vi "Main - Stock Ticker.vi"() -> ()   [LabVIEW 2011]
doc: "Main VI for a stock ticker application.\n\nInstructions:\n1) Select the data source.\n2) Enter the stock's symbol. Note that, for every letter typed, an HTTP query is sent (this is a trade-off between expecting the user to know the quotes and using a local list of quotes).\n3) Press the add button to add the ticker to the stock table.\n4) Press the delete button to delete the ticker the stock table.\n5) The delay between quote refresh is adjustable.\n6) The stop button will stop the application."
panel:
  in  "Delete":bool
  out "Stock Table":string[][](table)
  in  "Source":enum16{"Google", "Yahoo"}(ring)
  out "Consumer":bool
  out "Producer":bool
  out "Timer":bool
  out "Updating":bool
  in  "Refresh":i32=5 caption="Refresh rate [s]" min=0
  in  "Stop":bool
  in  "Add":bool
  in  "Stock Data":T1
  out "error out":errorcluster
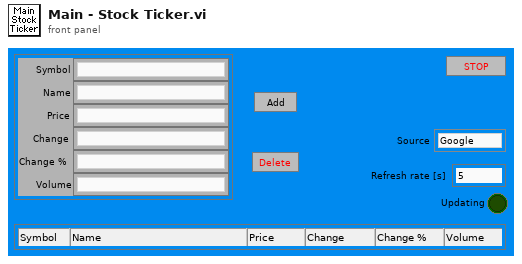
[diagram p1: front panel]
types:
  T1 = cluster{"Symbol":string, "Name":string, "Price":string, "Change":string, "Change %":string, "Volume":string}
  T2 = typedef "Queue RefNum" = refnum<k1>
  T3 = enum16{"Symbol", "Name", "Price", "Change", "Change %", "Volume"}
  T4 = typedef "Stock Data Control.ctl" = cluster{"Symbol":string, "Name":string, "Price":string, "Change":string, "Change %":string, "Volume":string}
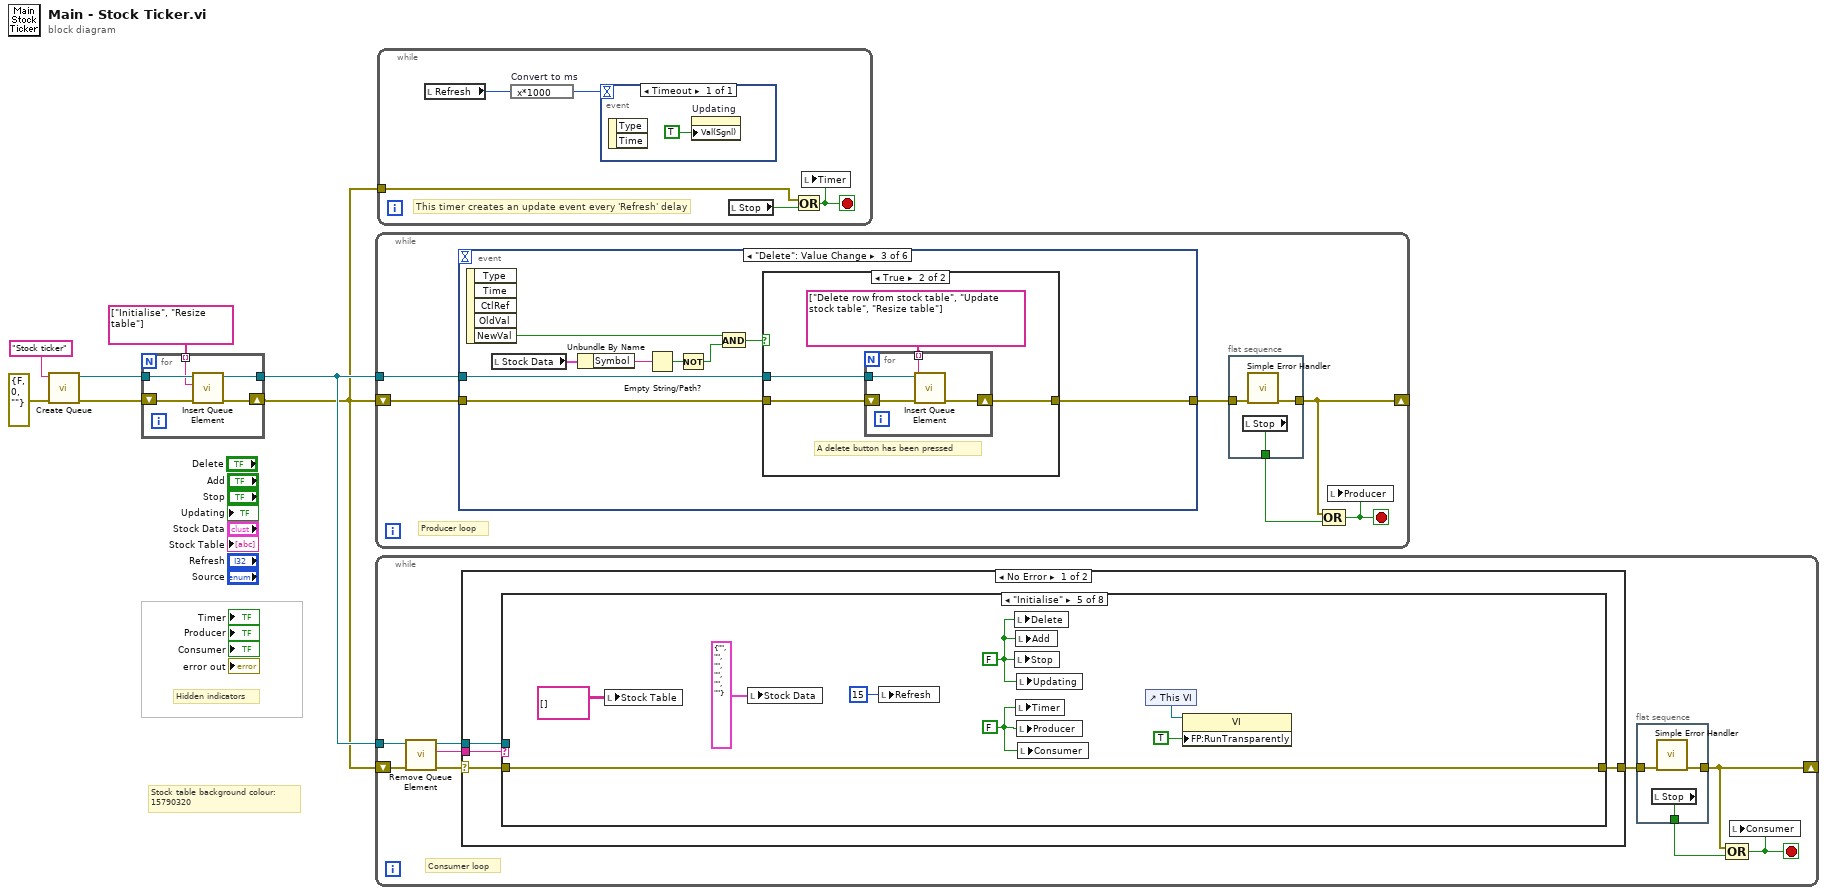
[diagram p0: block diagram]
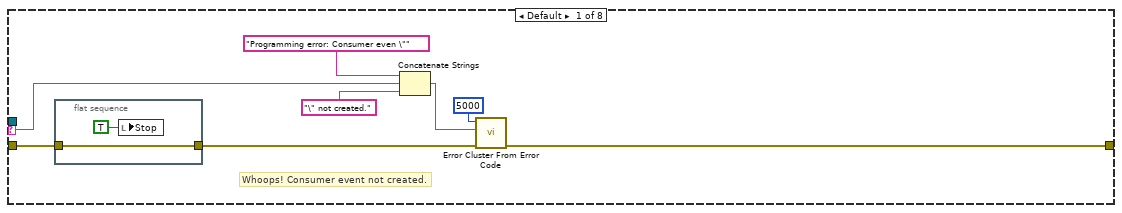
[diagram p2: hidden frame]
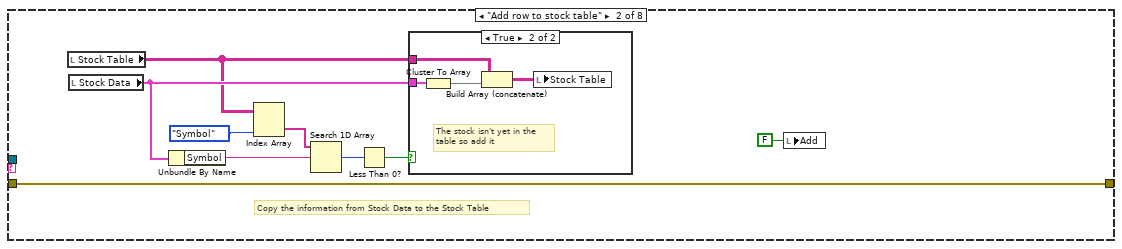
[diagram p3: hidden frame]
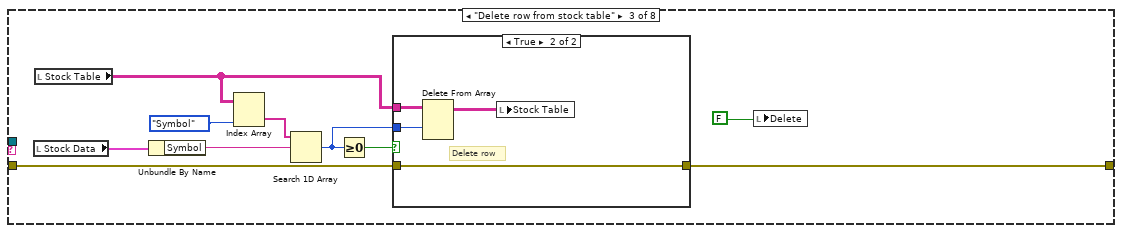
[diagram p5: hidden frame]
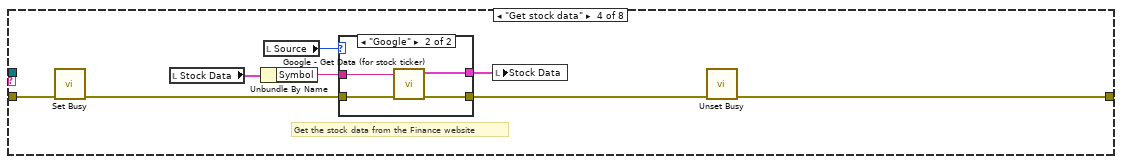
[diagram p7: hidden frame]
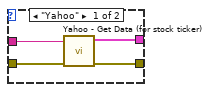
[diagram p8: hidden frame]
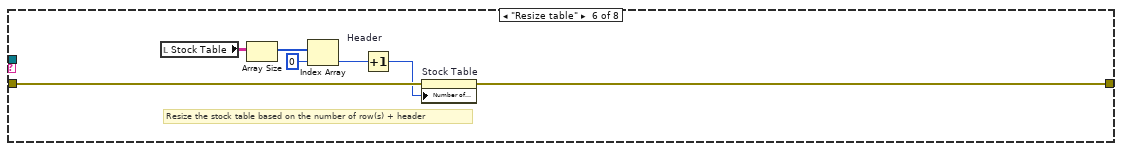
[diagram p9: hidden frame]
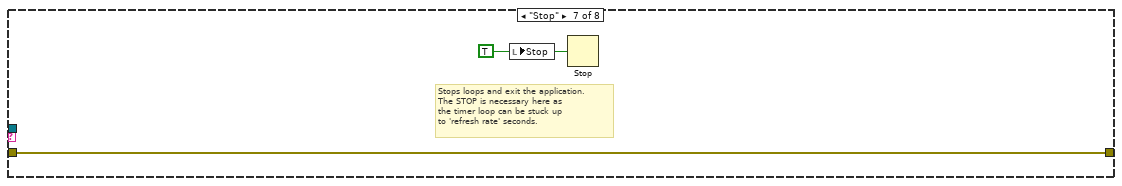
[diagram p10: hidden frame]
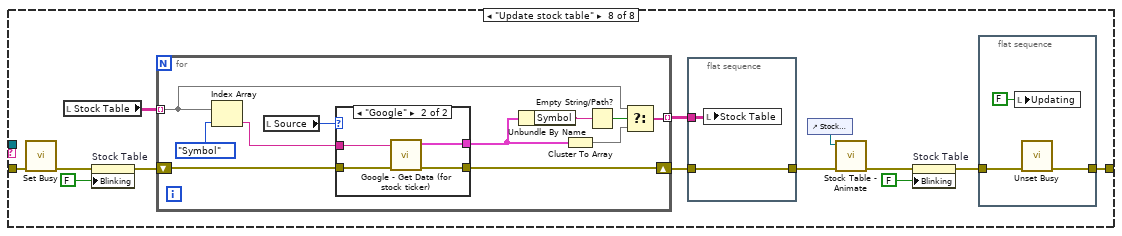
[diagram p11: hidden frame]
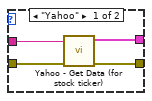
[diagram p12: hidden frame]
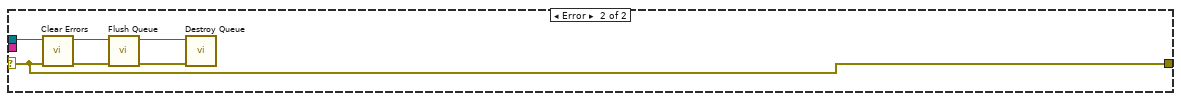
[diagram p13: hidden frame]
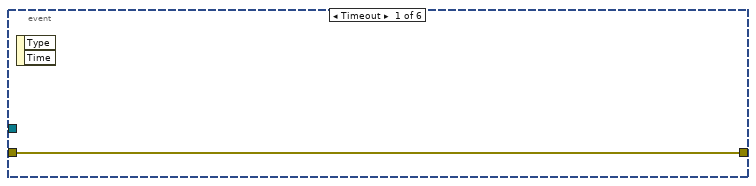
[diagram p14: hidden frame]
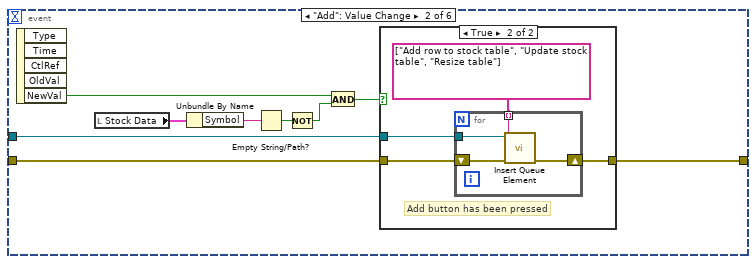
[diagram p15: hidden frame]
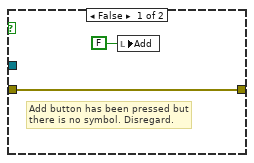
[diagram p16: hidden frame]
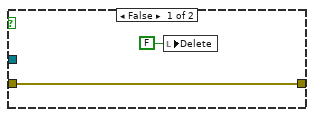
[diagram p17: hidden frame]
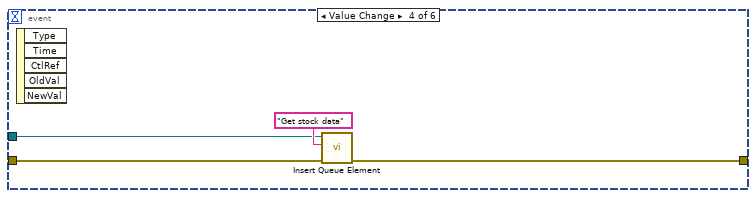
[diagram p18: hidden frame]
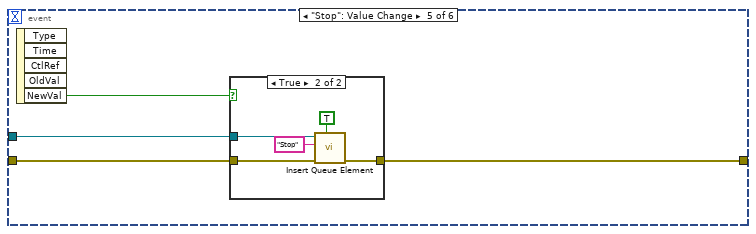
[diagram p19: hidden frame]
diagram:
  # "Stock table background colour:\n15790320"
  # "Hidden indicators"
  n1 = call <vilib>:"Create Queue.vi"("error in (no error)"=errorcluster {"status"=FALSE, "code"=0, "source"=""} ("error in"), "name (unnamed)"="Stock ticker") -> ("error out"=w3:errorcluster, "queue out"=w5:T2)  [unwired: 3 in, 1 out]
  n2 = for {
    tunnel: w5 -> [w12]
    tunnel: [w11] -> w4
    tunnel: string[] ["Initialise", "Resize table"] -> [w10] mode=indexing
    shift-right: [w8] -> w1
    shift-left: w3 -> [w9]
    n3 = call <vilib>:"Insert Queue Element.vi"("error in (no error)"=w9, "queue element"=w10, "queue"=w12) -> ("error out"=w8:errorcluster, "queue out"=w11:T2)  [unwired: 4 in, 1 out]
  }
  n4 = while {
    shift-right: [w18] -> _
    shift-left: w1 -> [w17]
    tunnel: w4 -> [w15]
    stop <- w13 stop-if-true
    # "Producer loop"
    n5 = event shown="[2] \"Delete\": Value Change" {
      selector: _ -> [_ _ _ _ _ _]
      dyn-events: _ -> [_ _ _ _ _ _]
      timeout: _ -> [_ _ _ _ _ _]
      tunnel: w17 -> [w22 w30 w50 w63 w68 w86]
      tunnel: [w22 w31 w49 w62 w67 w84] -> w16
      tunnel: w15 -> [_ w29 w48 w61 w66 w83]
      event Timeout {
        n6 = event-data() -> ()  [unwired: 1 in, 2 out]
      }
      event "Add": Value Change {
        n7 = event-data() -> ("NewVal"=w23:bool)  [unwired: 1 in, 4 out]
        n8 = local read "Stock Data"() -> (w27:T1)
        n9 = Unbundle By Name(w27) -> ("Symbol"=w26:string)
        n10 = Empty String/Path?(string/path=w26) -> (empty?=w25:bool)
        n11 = Not(x=w25) -> (.not. x?=w24:bool)
        n12 = And(x=w23, y=w24) -> (x .and. y?=w28:bool)
        n13 = case shown="True" w28 {
          tunnel: w30 -> [w33 w36]
          tunnel: [w33 w35] -> w31
          tunnel: w29 -> [_ w34]
          frame False {
            # "Add button has been pressed but\nthere is no symbol. Disregard."
            n14 = local write "Add"(FALSE ("Add")) -> ()
          }
          frame True {
            # "Add button has been pressed"
            n15 = for {
              tunnel: string[] ["Add row to stock table", "Update stock table", "Resize table"] -> [w41] mode=indexing
              shift-right: [w39] -> w35
              shift-left: w36 -> [w40]
              tunnel: w34 -> [w38]
              n16 = call <vilib>:"Insert Queue Element.vi"("error in (no error)"=w40, "queue element"=w41, "queue"=w38) -> ("error out"=w39:errorcluster)  [unwired: 4 in, 2 out]
            }
          }
        }
      }
      event "Delete": Value Change {
        n17 = event-data() -> ("NewVal"=w43:bool)  [unwired: 1 in, 4 out]
        n18 = local read "Stock Data"() -> (w42:T1)
        n19 = Unbundle By Name(w42) -> ("Symbol"=w47:string)
        n20 = Empty String/Path?(string/path=w47) -> (empty?=w46:bool)
        n21 = Not(x=w46) -> (.not. x?=w45:bool)
        n22 = And(x=w43, y=w45) -> (x .and. y?=w44:bool)
        n23 = case shown="True" w44 {
          tunnel: w50 -> [w52 w56]
          tunnel: [w52 w55] -> w49
          tunnel: w48 -> [_ w54]
          frame False {
            n24 = local write "Delete"(FALSE ("Delete")) -> ()
          }
          frame True {
            # "A delete button has been pressed"
            n25 = for {
              tunnel: string[] ["Delete row from stock table", "Update stock table", "Resize table"] -> [w60] mode=indexing
              shift-right: [w58] -> w55
              shift-left: w56 -> [w59]
              tunnel: w54 -> [w57]
              n26 = call <vilib>:"Insert Queue Element.vi"("error in (no error)"=w59, "queue element"=w60, "queue"=w57) -> ("error out"=w58:errorcluster)  [unwired: 4 in, 2 out]
            }
          }
        }
      }
      event "Stock Data.Symbol": Value Change {
        n27 = event-data() -> ()  [unwired: 1 in, 5 out]
        n28 = call <vilib>:"Insert Queue Element.vi"("error in (no error)"=w63, "queue element"="Get stock data", "queue"=w61) -> ("error out"=w62:errorcluster)  [unwired: 4 in, 2 out]
      }
      event "Stop": Value Change {
        n29 = event-data() -> ("NewVal"=w65:bool)  [unwired: 1 in, 4 out]
        n30 = case shown="True" w65 {
          tunnel: w68 -> [w69 w74]
          tunnel: [w69 w73] -> w67
          tunnel: w66 -> [_ w71]
          frame False {
          }
          frame True {
            n31 = call <vilib>:"Insert Queue Element.vi"("at front (F)"=TRUE, "error in (no error)"=w74, "queue element"="Stop", "queue"=w71) -> ("error out"=w73:errorcluster)  [unwired: 3 in, 2 out]
          }
        }
      }
      event "Updating": Value Change {
        # "1+2)  Sequence OFF->ON\n3) # of pending elements = 0\n4) # of queue elements = 0"
        n32 = event-data() -> ("OldVal"=w75:bool, "NewVal"=w76:bool)  [unwired: 1 in, 3 out]
        n33 = call <vilib>:"Get Queue Status.vi"("error in (no error)"=w86, "queue"=w83) -> ("error out"=w85:errorcluster, "# pending to insert"=w81:i32, "queue out"=w77:T2, "# elements in queue"=w82:i32)  [unwired: 2 in, 4 out]
        n34 = Equal To 0?(x=w82) -> (x = 0?=w79:bool)
        n35 = Equal To 0?(x=w81) -> (x = 0?=w80:bool)
        n36 = Compound Arithmetic op=AND(invert w75, w76, w80, w79) -> (w78:bool)
        n37 = case shown="True" w78 {
          tunnel: w85 -> [w87 w90]
          tunnel: [w87 w89] -> w84
          tunnel: w77 -> [_ w88]
          frame False {
          }
          frame True {
            # "Time to update the stock table"
            n38 = call <vilib>:"Insert Queue Element.vi"("error in (no error)"=w90, "queue element"="Update stock table", "queue"=w88) -> ("error out"=w89:errorcluster)  [unwired: 4 in, 2 out]
          }
        }
      }
    }
    n39 = flat-sequence {
      tunnel: [w21] -> w18
      tunnel: w16 -> [w20]
      tunnel: [w19] -> w14
      frame #0 {
        n40 = local read "Stop"() -> (w19:bool)
        n41 = call <vilib>:"Simple Error Handler.vi"("error in (no error)"=w20) -> ("error out"=w21:errorcluster)  [unwired: 4 in, 4 out]
      }
    }
    n42 = Compound Arithmetic op=OR(w18, w14) -> (w13:bool)
    n43 = local write "Producer"(w13) -> ()
  }
  n44 = while {
    tunnel: w4 -> [w100]
    shift-right: [w94] -> _
    shift-left: w1 -> [w99]
    stop <- w92 stop-if-true
    # "Consumer loop"
    n45 = call <vilib>:"Remove Queue Element.vi"("error in (no error)"=w99, "queue"=w100) -> ("error out"=w98:errorcluster, "queue element"=w97:string, "queue out"=w95:T2)  [unwired: 4 in, 1 out]
    n46 = case shown="No Error" w98 {
      selector: w98 -> [w106 w217]
      tunnel: [w105 w217] -> w96
      tunnel: w97 -> [w107 _]
      tunnel: w95 -> [w104 w216]
      frame No Error {
        n47 = case shown="\"Initialise\"" w107 {
          selector: w107 -> [w113 _ _ _ _ _ _ _]
          tunnel: w106 -> [w109 w125 w133 w151 w169 w176 w178 w189]
          tunnel: [w110 w125 w132 w152 w169 w175 w178 w190] -> w105
          tunnel: w104 -> [_ _ _ _ _ _ _ _]
          frame Default {
            # "Whoops! Consumer event not created."
            n48 = flat-sequence {
              tunnel: w109 -> [w116]
              tunnel: [w116] -> w108
              frame #0 {
                n49 = local write "Stop"(TRUE ("Stop")) -> ()
              }
            }
            n50 = Concatenate Strings("Programming error: Consumer even \"" ("error message (\"\")"), w113, "\" not created.") -> (w115:string)
            n51 = call <vilib>:"Error Cluster From Error Code.vi"("error in (no error)"=w108, "error message (\"\")"=w115, "error code (0)"=5000) -> ("error out"=w110:errorcluster)  [unwired: 6 in]
          }
          frame "Add row to stock table" {
            # "Copy the information from Stock Data to the Stock Table"
            n52 = local read "Stock Table"() -> (w123:string[][])
            n53 = local read "Stock Data"() -> (w124:T1)
            n54 = Unbundle By Name(w124) -> ("Symbol"=w120:string)
            n55 = Index Array(array=w123, index (col)=T3."Symbol") -> (element=w121:string[])  [unwired: 1 in]
            n56 = Search 1D Array(1D array=w121, element=w120) -> (index of element=w119:i32)  [unwired: 1 in]
            n57 = Less Than 0?(x=w119) -> (x < 0?=w118:bool)
            n58 = case shown="True" w118 {
              tunnel: w124 -> [_ w128]
              tunnel: w123 -> [_ w127]
              frame False {
                # "Stock already in the table.\nNo duplicate allowed."
              }
              frame True {
                # "The stock isn't yet in the\ntable so add it"
                n59 = Cluster To Array(cluster=w128) -> (array=w129:string[])
                n60 = Build Array (concatenate)(w127, w129) -> (w130:string[][])
                n61 = local write "Stock Table"(w130) -> ()
              }
            }
            n62 = local write "Add"(FALSE ("Add")) -> ()
          }
          frame "Delete row from stock table" {
            n63 = local read "Stock Data"() -> (w137:T1)
            n64 = local read "Stock Table"() -> (w134:string[][])
            n65 = Unbundle By Name(w137) -> ("Symbol"=w138:string)
            n66 = Index Array(array=w134, index (col)=T3."Symbol") -> (element=w139:string[])  [unwired: 1 in]
            n67 = Search 1D Array(1D array=w139, element=w138) -> (index of element=w135:i32)  [unwired: 1 in]
            n68 = Greater Or Equal To 0?(x=w135) -> (x >= 0?=w136:bool)
            n69 = case shown="True" w136 {
              tunnel: w135 -> [_ w144]
              tunnel: w134 -> [_ w143]
              tunnel: w133 -> [w141 w142]
              tunnel: [w141 w142] -> w132
              frame False {
                # "Nothing to delete"
              }
              frame True {
                # "Delete row"
                n70 = Delete From Array(array=w143, index (row)=w144) -> (array with subset deleted=w145:string[][])  [unwired: 2 in, 1 out]
                n71 = local write "Stock Table"(w145) -> ()
              }
            }
            n72 = local write "Delete"(FALSE ("Delete")) -> ()
          }
          frame "Get stock data" {
            # "Get the stock data from the Finance website"
            n73 = call <vilib>:"Set Busy.vi"("error in (no error)"=w151) -> ("error out"=w148:errorcluster)  [unwired: 9 in, 1 out]
            n74 = local read "Stock Data"() -> (w153:T1)
            n75 = Unbundle By Name(w153) -> ("Symbol"=w149:string)
            n76 = local read "Source"() -> (w150:enum16{"Google", "Yahoo"})
            n77 = case shown="\"Google\"" w150 {
              tunnel: w148 -> [w157 w161]
              tunnel: [w155 w159] -> w147
              tunnel: [w154 w158] -> w146
              tunnel: w149 -> [w156 w160]
              frame "Yahoo" {
                n78 = call "Yahoo - Get Data (for stock ticker).vi"("Symbol"=w156, "error in"=w157) -> ("Stock Data"=w154:T4, "error out"=w155:errorcluster)  [unwired: 6 in]
              }
              frame "Google" {
                n79 = call "Google - Get Data (for stock ticker).vi"("Symbol"=w160, "error in"=w161) -> ("Stock Data"=w158:T4, "error out"=w159:errorcluster)  [unwired: 6 in]
              }
            }
            n80 = local write "Stock Data"(w146) -> ()
            n81 = call <vilib>:"Unset Busy.vi"("error in (no error)"=w147) -> ("error out"=w152:errorcluster)  [unwired: 10 in]
          }
          frame "Initialise" {
            w165 = FALSE ("stop")
            w162 = FALSE ("stop")
            n82 = local write "Stock Table"(string[][] [] ("Stock array")) -> ()
            n83 = local write "Stock Data"(T1 {"Symbol"="", "Name"="", "Price"="", "Change"="", "Change %"="", "Volume"=""} ("Stock Data")) -> ()
            n84 = local write "Refresh"(15 ("Refresh")) -> ()
            n85 = local write "Delete"(w162) -> ()
            n86 = local write "Stop"(w162) -> ()
            n87 = local write "Add"(w162) -> ()
            n88 = local write "Timer"(w165) -> ()
            n89 = local write "Updating"(w162) -> ()
            n90 = local write "Producer"(w165) -> ()
            n91 = local write "Consumer"(w165) -> ()
            n92 = control-ref of="This VI"() -> (w163:refnum<vi>)
            n93 = property on="Property Node" class="VI"(reference=w163, "FP:RunTransparently"=TRUE ("Front Panel Window:Run VI Transparently")) -> ()  [unwired: 1 in, 2 out]
          }
          frame "Resize table" {
            # "Resize the stock table based on the number of row(s) + header"
            n94 = local read "Stock Table"() -> (w174:string[][])
            n95 = Array Size(array=w174) -> (size(s)=w173:i32[])
            n96 = Index Array(array=w173, index=0) -> (element=w171:i32)
            n97 = Increment "Header"(x=w171) -> (x+1=w170:i32)
            n98 = property on="Stock Table" class="Tbl (strict)"(error in=w176, "Number of Rows"=w170) -> (error out=w175:errorcluster)  [unwired: 1 in, 1 out]
          }
          frame "Stop" {
            w177 = TRUE ("stop")
            # "Stops loops and exit the application.\nThe STOP is necessary here as\nthe timer loop can be stuck up\nto 'refresh rate' seconds."
            n99 = local write "Stop"(w177) -> ()
            n100 = Stop(stop? (T)=w177) -> ()
          }
          frame "Update stock table" {
            n101 = call <vilib>:"Set Busy.vi"("error in (no error)"=w189) -> ("error out"=w186:errorcluster)  [unwired: 9 in, 1 out]
            n102 = local read "Stock Table"() -> (w188:string[][])
            n103 = property on="Stock Table" class="Tbl (strict)"(error in=w186, "Blinking"=FALSE ("Synchronous Display")) -> (error out=w185:errorcluster)  [unwired: 1 in, 1 out]
            n104 = for {
              shift-right: [w206] -> w180
              shift-left: w185 -> [w207]
              tunnel: [w198] -> w191 mode=indexing
              tunnel: w188 -> [w200] mode=indexing
              n105 = Index Array(array=w200, index=T3."Symbol") -> (element=w203:string)
              n106 = local read "Source"() -> (w197:enum16{"Google", "Yahoo"})
              n107 = case shown="\"Google\"" w197 {
                tunnel: w207 -> [w211 w215]
                tunnel: [w209 w213] -> w206
                tunnel: [w208 w212] -> w205
                tunnel: w203 -> [w210 w214]
                frame "Yahoo" {
                  n108 = call "Yahoo - Get Data (for stock ticker).vi"("Symbol"=w210, "error in"=w211) -> ("Stock Data"=w208:T4, "error out"=w209:errorcluster)  [unwired: 6 in]
                }
                frame "Google" {
                  n109 = call "Google - Get Data (for stock ticker).vi"("Symbol"=w214, "error in"=w215) -> ("Stock Data"=w212:T4, "error out"=w213:errorcluster)  [unwired: 6 in]
                }
              }
              n110 = Unbundle By Name(w205) -> ("Symbol"=w204:string)
              n111 = Cluster To Array(cluster=w205) -> (array=w199:string[])
              n112 = Empty String/Path?(string/path=w204) -> (empty?=w201:bool)
              n113 = Select(t=w200, s=w201, f=w199) -> (s? t:f=w198:string[])
            }
            n114 = flat-sequence {
              tunnel: w191 -> [w193]
              tunnel: w180 -> [w192]
              tunnel: [w192] -> w179
              frame #0 {
                n115 = local write "Stock Table"(w193) -> ()
              }
            }
            n116 = control-ref of="Stock Table"() -> (w187:refnum<vi>)
            n117 = call "Stock Table - Animate.vi"("error in"=w179, "Table Reference"=w187) -> ("error out"=w183:errorcluster)  [unwired: 9 in]
            n118 = property on="Stock Table" class="Tbl (strict)"(error in=w183, "Blinking"=FALSE ("Synchronous Display")) -> (error out=w182:errorcluster)  [unwired: 1 in, 1 out]
            n119 = flat-sequence {
              tunnel: [w195] -> w190
              tunnel: w182 -> [w194]
              frame #0 {
                n120 = local write "Updating"(FALSE ("Update")) -> ()
                n121 = call <vilib>:"Unset Busy.vi"("error in (no error)"=w194) -> ("error out"=w195:errorcluster)  [unwired: 10 in]
              }
            }
          }
        }
      }
      frame Error {
        n122 = call <vilib>:"Clear Errors.vi"("error in (no error)"=w217) -> ()  [unwired: 6 in, 1 out]
        n123 = call <vilib>:"Flush Queue.vi"("error in (no error)"=w217, "queue"=w216) -> ("error out"=w219:errorcluster, "queue out"=w218:T2)  [unwired: 3 in, 1 out]
        n124 = call <vilib>:"Destroy Queue.vi"("error in (no error)"=w219, "queue"=w218) -> ()  [unwired: 3 in, 3 out]
      }
    }
    n125 = flat-sequence {
      tunnel: w96 -> [w103]
      tunnel: [w102] -> w93
      tunnel: [w101] -> w94
      frame #0 {
        n126 = local read "Stop"() -> (w102:bool)
        n127 = call <vilib>:"Simple Error Handler.vi"("error in (no error)"=w103) -> ("error out"=w101:errorcluster)  [unwired: 4 in, 4 out]
      }
    }
    n128 = Compound Arithmetic op=OR(w94, w93) -> (w92:bool)
    n129 = local write "Consumer"(w92) -> ()
  }
  n130 = while {
    tunnel: w1 -> [w224]
    stop <- w222 stop-if-true
    # "This timer creates an update event every 'Refresh' delay"
    n131 = local read "Refresh"() -> (w220:i32)
    n132 = expression code="x*1000" "Convert to ms"(w220) -> (w221:i32)
    n133 = event shown="[0] Timeout" {
      selector: _ -> [_]
      dyn-events: _ -> [_]
      timeout: w221 -> [_]
      event Timeout {
        n134 = event-data() -> ()  [unwired: 1 in, 2 out]
        n135 = property on="Updating" class="Bool (strict)"("Val(Sgnl)"=TRUE ("Value (Signaling)")) -> ()  [unwired: 2 in, 2 out]
      }
    }
    n136 = local read "Stop"() -> (w223:bool)
    n137 = Or(x=w224, y=w223) -> (x .or. y?=w222:bool)
    n138 = local write "Timer"(w222) -> ()
  }
